vi "UARTTestTx.vi"(7 "device":string, 8 "error in (no error)":errorcluster, 9 "value":string, 10 "method":string, 11 "Sequence Context In":refnum<k7>) -> (0 "error out":errorcluster, 2 "status":string)   [LabVIEW 2021]
uses:
  <vilib>/addons/TestStand/_TSUtility.llb/TestStand - Get Property Value (String).vi
  <vilib>/NI/JSON Support for LabVIEW/JSON Value/New JSON Value/New JSON ({String}).vi
  <vilib>/NI/JSON Support for LabVIEW/JSON Value/Object/Insert Value/Insert Value (String).vi
  <vilib>/NI/NI JSONRPC Server Framework/Classes/Client/Format Client Request (Auto-Increment).vi
  <vilib>/NI/JSON Support for LabVIEW/JSON Value/JSON Value.lvclass
  <vilib>/NI/NI JSONRPC Server Framework/Classes/Client/JSONRPC Client.lvclass
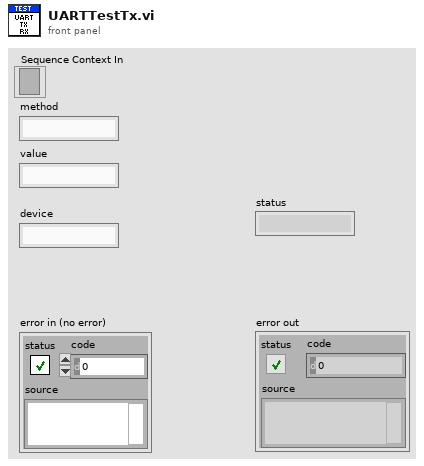
[diagram p1: front panel]
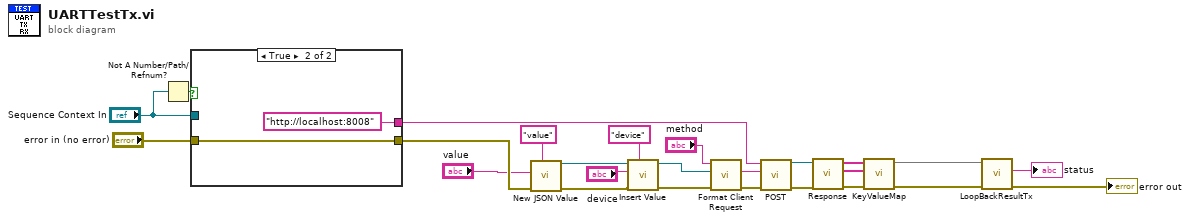
[diagram p0: block diagram]
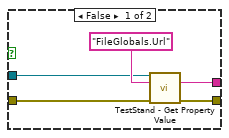
[diagram p2: hidden frame]
diagram:
  n1 = Not A Number/Path/Refnum?(number/path/refnum="Sequence Context In") -> (NaN/Path/Refnum?=w10:bool)
  n2 = case shown="True" w10 {
    tunnel: [w29 "http://localhost:8008" ("Value")] -> w25
    tunnel: [w28 w31] -> w4
    tunnel: "error in (no error)" -> [w27 w31]
    tunnel: "Sequence Context In" -> [w26 _]
    frame False {
      n3 = call-poly <vilib>:"TestStand - Get Property Value.vi"("Sequence Context In"=w26, "Lookup String"="FileGlobals.Url", "error in (no error)"=w27) -> ("Value"=w29:string, "error out"=w28:errorcluster)  [unwired: 10 in, 1 out]
    }
    frame True {
    }
  }
  n4 = call-poly <vilib>:"New JSON Value.vi"("key"="value", "error in (no error)"=w4, "value"="value") -> ("error out"=w9:errorcluster, "JSON Value out"=w8:refnum<class "JSON Value.lvclass">)  [unwired: 7 in]
  n5 = call-poly <vilib>:"Insert Value.vi"("key"="device", "error in (no error)"=w9, "value"="device", "JSON Value in"=w8) -> ("error out"=w3:errorcluster, "JSON Value out"=w1:refnum<class "JSON Value.lvclass">)  [unwired: 5 in, 1 out]
  n6 = call-poly <vilib>:"Format Client Request.vi"("error in (no error)"=w3, "JSON Value in"=w1, "method"="method") -> ("error out"=w16:errorcluster, "Request String"=w17:string)  [unwired: 7 in]
  n7 = call "POST.vi"("error in (no error)"=w16, "Request String"=w17, "url"=w25) -> ("error out"=w18:errorcluster, "JSON Value out"=w19:refnum<class "JSON Value.lvclass">)  [unwired: 7 in]
  n8 = call "Response.vi"("error in (no error)"=w18, "JSON Value in"=w19) -> ("error out"=w20:errorcluster, "values"=w22:string[], "keys"=w21:string[])  [unwired: 7 in]
  n9 = call "KeyValueMap.vi"("error in"=w20, "values"=w22, "keys"=w21) -> ("error out"=w13:errorcluster, "map out"=w14:map{string, string})  [unwired: 7 in]
  n10 = call "LoopBackResultTx.vi"("error in (no error)"=w13, "map"=w14) -> ("error out"=→"error out":errorcluster, "status"=→"status":string)  [unwired: 8 in]
